vi "Frequency Linearization SubVI.vi"(8 "Scale factor":dbl(slide)=0.5 scale=0.01..1.0, 9 "#Medie":i32=20, 10 "Sketri Input":dbl[](array[numeric])=[2047.0, 2034.0, 2021.0, 2008.0, 1995.0, 1982.0, 1969.0, 1956.0, 1943.0, 1930.0, 1917.0, 1904.0, 1891.0, 1879.0, 1866.0, 1853.0, 1840.0, 1827.0, 1815.0, 1802.0, 1789.0, 1777.0, 1764.0, 1751.0, 1739.0, 1726.0, 1714.0, 1701.0, 1689.0, 1676.0, 1664.0, 1651.0, 1639.0, 1626.0, 1614.0, 1602.0, 1589.0, 1577.0, 1565.0, 1552.0, 1540.0, 1528.0, 1516.0, 1503.0, 1491.0, 1479.0, 1467.0, 1455.0, 1443.0, 1431.0, 1419.0, 1407.0, 1395.0, 1383.0, 1371.0, 1359.0, 1347.0, 1335.0, 1323.0, 1311.0, 1299.0, 1287.0, 1276.0, 1264.0, 1252.0, 1240.0, 1229.0, 1217.0, 1205.0, 1194.0, 1182.0, 1170.0, 1159.0, 1147.0, 1136.0, 1124.0, 1113.0, 1101.0, 1090.0, 1078.0, 1067.0, 1055.0, 1044.0, 1033.0, 1021.0, 1010.0, 999.0, 987.0, 976.0, 965.0, 954.0, 942.0, 931.0, 920.0, 909.0, 898.0, 887.0, 876.0, 865.0, 854.0, 843.0, 832.0, 821.0, 810.0, 799.0, 788.0, 777.0, 766.0, 755.0, 744.0, 734.0, 723.0, 712.0, 701.0, 691.0, 685.0, 679.0, 674.0, 665.0, 658.0, 652.0, 647.0, 640.0, 634.0, 628.0, 618.0, 612.0, 605.0, 600.0, 594.0, 587.0, 582.0, 575.0, 570.0, 564.0, 559.0, 553.0, 548.0, 542.0, 537.0, 531.0, 525.0, 520.0, 514.0, 509.0, 503.0, 497.0, 492.0, 486.0, 480.0, 475.0, 469.0, 463.0, 458.0, 452.0, 446.0, 441.0, 435.0, 429.0, 423.0, 417.0, 411.0, 406.0, 400.0, 395.0, 389.0, 383.0, 377.0, 372.0, 366.0, 360.0, 355.0, 349.0, 344.0, 338.0, 333.0, 328.0, 322.0, 317.0, 311.0, 306.0, 300.0, 295.0, 289.0, 284.0, 278.0, 273.0, 268.0, 262.0, 257.0, 251.0, 246.0, 240.0, 235.0, 229.0, 224.0, 219.0, 213.0, 208.0, 202.0, 197.0, 191.0, 186.0, 181.0, 175.0, 170.0, 164.0, 159.0, 154.0, 148.0, 143.0, 137.0, 132.0, 127.0, 121.0, 116.0, 110.0, 105.0, 100.0, 94.0, 89.0, 84.0, 78.0, 73.0, 67.0, 62.0, 57.0, 51.0, 46.0, 41.0, 35.0, 30.0, 25.0, 19.0, 14.0, 8.0, 3.0, -3.0, -8.0, -13.0, -18.0, -24.0, -29.0, -35.0, -40.0, -45.0, -51.0, -56.0, -62.0, -67.0, -72.0, -78.0, -83.0, -88.0, -94.0, -99.0, -104.0, -110.0, -115.0, -120.0, -126.0, -131.0, -137.0, -142.0, -147.0, -153.0, -158.0, -163.0, -169.0, -174.0, -179.0, -185.0, -190.0, -195.0, -201.0, -206.0, -211.0, -217.0, -222.0, -227.0, -233.0, -238.0, -243.0, -249.0, -254.0, -259.0, -265.0, -270.0, -275.0, -281.0, -286.0, -291.0, -297.0, -302.0, -307.0, -313.0, -318.0, -323.0, -329.0, -334.0, -339.0, -345.0, -350.0, -355.0, -361.0, -366.0, -371.0, -377.0, -382.0, -387.0, -393.0, -398.0, -403.0, -408.0, -414.0, -419.0, -424.0, -430.0, -435.0, -440.0, -446.0, -451.0, -456.0, -462.0, -467.0, -472.0, -478.0, -483.0, -488.0, -494.0, -499.0, -504.0, -510.0, -515.0, -520.0, -526.0, -531.0, -536.0, -541.0, -547.0, -552.0, -557.0, -563.0, -568.0, -573.0, -579.0, -584.0, -589.0, -594.0, -600.0, -605.0, -610.0, -616.0, -621.0, -626.0, -631.0, -637.0, -642.0, -647.0, -652.0, -658.0, -663.0, -668.0, -673.0, -679.0, -684.0, -689.0, -695.0, -700.0, -705.0, -710.0, -716.0, -721.0, -726.0, -731.0, -737.0, -742.0, -747.0, -753.0, -758.0, -763.0, -768.0, -774.0, -779.0, -784.0, -789.0, -795.0, -800.0, -805.0, -811.0, -816.0, -821.0, -826.0, -832.0, -837.0, -842.0, -848.0, -853.0, -858.0, -864.0, -869.0, -874.0, -879.0, -885.0, -890.0, -895.0, -901.0, -906.0, -911.0, -916.0, -922.0, -927.0, -932.0, -938.0, -943.0, -948.0, -953.0, -959.0, -964.0, -969.0, -974.0, -980.0, -985.0, -990.0, -996.0, -1001.0, -1006.0, -1011.0, -1017.0, -1022.0, -1027.0, -1032.0, -1038.0, -1043.0, -1048.0, -1054.0, -1059.0, -1064.0, -1069.0, -1075.0, -1080.0, -1085.0, -1090.0, -1096.0, -1101.0, -1106.0, -1112.0, -1117.0, -1122.0, -1127.0, -1133.0, -1138.0, -1143.0, -1148.0, -1154.0, -1159.0, -1164.0, -1169.0, -1175.0, -1180.0, -1185.0, -1191.0, -1196.0, -1201.0, -1206.0, -1212.0, -1217.0, -1222.0, -1227.0, -1233.0, -1238.0, -1243.0, -1249.0, -1254.0, -1259.0, -1264.0, -1270.0, -1275.0, -1280.0, -1285.0, -1291.0, -1296.0, -1301.0, -1306.0, -1312.0, -1317.0, -1322.0, -1328.0, -1333.0, -1338.0, -1343.0, -1349.0, -1354.0, -1359.0, -1364.0, -1370.0, -1375.0, -1380.0, -1385.0, -1391.0, -1396.0, -1401.0, -1407.0, -1412.0, -1417.0, -1422.0, -1428.0, -1433.0, -1438.0, -1443.0, -1449.0, -1454.0, -1459.0, -1464.0, -1470.0, -1475.0, -1480.0, -1486.0, -1491.0, -1496.0, -1501.0, -1507.0, -1512.0, -1517.0, -1522.0, -1528.0, -1533.0, -1538.0, -1543.0, -1549.0, -1554.0, -1559.0, -1564.0, -1570.0, -1575.0, -1580.0, -1586.0, -1591.0, -1596.0, -1601.0, -1607.0, -1612.0, -1617.0, -1622.0, -1628.0, -1633.0, -1638.0, -1643.0, -1649.0, -1654.0, -1659.0, -1664.0, -1670.0, -1675.0, -1680.0, -1685.0, -1691.0, -1696.0, -1701.0, -1706.0, -1712.0, -1717.0, -1722.0, -1728.0, -1733.0, -1738.0, -1743.0, -1749.0, -1754.0, -1759.0, -1764.0, -1770.0, -1775.0, -1780.0, -1785.0, -1791.0, -1796.0, -1801.0, -1806.0, -1812.0, -1817.0, -1822.0, -1827.0, -1833.0, -1838.0, -1843.0, -1848.0, -1854.0, -1859.0, -1864.0, -1869.0, -1875.0, -1880.0, -1885.0, -1890.0, -1896.0, -1901.0, -1906.0, -1911.0, -1917.0, -1922.0, -1927.0, -1932.0, -1938.0, -1943.0, -1948.0, -1953.0, -1959.0, -1964.0, -1969.0, -1974.0, -1980.0, -1985.0, -1990.0, -1995.0, -2001.0, -2006.0, -2011.0, -2016.0, -2022.0, -2027.0, -2032.0, -2037.0, -2043.0, -2048.0, -2047.0, -2037.0, -2028.0, -2018.0, -2008.0, -1999.0, -1989.0, -1979.0, -1970.0, -1960.0, -1951.0, -1941.0, -1931.0, -1922.0, -1912.0, -1903.0, -1893.0, -1884.0, -1874.0, -1865.0, -1855.0, -1846.0, -1836.0, -1827.0, -1817.0, -1808.0, -1798.0, -1789.0, -1779.0, -1770.0, -1761.0, -1751.0, -1742.0, -1732.0, -1723.0, -1714.0, -1704.0, -1695.0, -1686.0, -1676.0, -1667.0, -1658.0, -1648.0, -1639.0, -1630.0, -1621.0, -1611.0, -1602.0, -1593.0, -1584.0, -1575.0, -1565.0, -1556.0, -1547.0, -1538.0, -1529.0, -1520.0, -1510.0, -1501.0, -1492.0, -1483.0, -1474.0, -1465.0, -1456.0, -1447.0, -1438.0, -1429.0, -1420.0, -1411.0, -1402.0, -1393.0, -1384.0, -1375.0, -1366.0, -1357.0, -1348.0, -1339.0, -1330.0, -1321.0, -1312.0, -1303.0, -1294.0, -1285.0, -1277.0, -1268.0, -1259.0, -1250.0, -1241.0, -1232.0, -1224.0, -1215.0, -1206.0, -1197.0, -1188.0, -1180.0, -1171.0, -1162.0, -1153.0, -1145.0, -1136.0, -1127.0, -1119.0, -1110.0, -1101.0, -1093.0, -1084.0, -1075.0, -1067.0, -1058.0, -1049.0, -1041.0, -1032.0, -1024.0, -1015.0, -1007.0, -998.0, -989.0, -981.0, -972.0, -964.0, -955.0, -909.0, -902.0, -894.0, -872.0, -865.0, -858.0, -850.0, -843.0, -836.0, -781.0, -774.0, -747.0, -740.0, -734.0, -727.0, -720.0, -714.0, -707.0, -700.0, -693.0, -687.0, -679.0, -672.0, -654.0, -647.0, -639.0, -632.0, -625.0, -619.0, -608.0, -601.0, -595.0, -588.0, -582.0, -575.0, -568.0, -562.0, -555.0, -549.0, -542.0, -535.0, -529.0, -522.0, -515.0, -509.0, -502.0, -496.0, -489.0, -482.0, -476.0, -469.0, -462.0, -456.0, -449.0, -441.0, -435.0, -427.0, -420.0, -413.0, -407.0, -401.0, -395.0, -387.0, -381.0, -373.0, -367.0, -361.0, -355.0, -349.0, -343.0, -337.0, -330.0, -324.0, -318.0, -312.0, -306.0, -300.0, -294.0, -288.0, -282.0, -276.0, -269.0, -263.0, -257.0, -251.0, -245.0, -239.0, -233.0, -227.0, -221.0, -215.0, -209.0, -203.0, -197.0, -191.0, -185.0, -179.0, -173.0, -167.0, -161.0, -155.0, -149.0, -143.0, -137.0, -131.0, -125.0, -119.0, -113.0, -107.0, -101.0, -95.0, -89.0, -83.0, -77.0, -71.0, -65.0, -59.0, -54.0, -48.0, -42.0, -36.0, -30.0, -23.0, -17.0, -11.0, -6.0, -0.0, 6.0, 13.0, 19.0, 25.0, 31.0, 37.0, 42.0, 48.0, 55.0, 61.0, 66.0, 72.0, 78.0, 84.0, 89.0, 95.0, 101.0, 106.0, 112.0, 118.0, 124.0, 129.0, 135.0, 141.0, 146.0, 152.0, 157.0, 163.0, 169.0, 174.0, 180.0, 186.0, 191.0, 197.0, 203.0, 208.0, 214.0, 219.0, 225.0, 231.0, 236.0, 242.0, 247.0, 253.0, 259.0, 264.0, 270.0, 275.0, 281.0, 287.0, 292.0, 298.0, 303.0, 309.0, 315.0, 320.0, 326.0, 331.0, 337.0, 343.0, 348.0, 354.0, 359.0, 365.0, 371.0, 376.0, 382.0, 387.0, 393.0, 399.0, 404.0, 410.0, 416.0, 421.0, 427.0, 433.0, 438.0, 444.0, 449.0, 455.0, 461.0, 466.0, 472.0, 477.0, 483.0, 488.0, 494.0, 500.0, 505.0, 511.0, 517.0, 522.0, 528.0, 533.0, 539.0, 544.0, 550.0, 555.0, 561.0, 566.0, 572.0, 577.0, 583.0, 588.0, 594.0, 599.0, 604.0, 610.0, 615.0, 621.0, 626.0, 632.0, 637.0, 643.0, 648.0, 654.0, 659.0, 665.0, 670.0, 675.0, 681.0, 686.0, 692.0, 697.0, 703.0, 708.0, 714.0, 719.0, 725.0, 730.0, 735.0, 741.0, 746.0, 752.0, 757.0, 763.0, 768.0, 774.0, 779.0, 785.0, 790.0, 795.0, 801.0, 806.0, 812.0, 817.0, 823.0, 828.0, 834.0, 839.0, 844.0, 850.0, 855.0, 861.0, 866.0, 872.0, 877.0, 882.0, 888.0, 893.0, 899.0, 904.0, 910.0, 915.0, 920.0, 926.0, 931.0, 937.0, 942.0, 947.0, 953.0, 958.0, 964.0, 969.0, 974.0, 980.0, 985.0, 991.0, 996.0, 1001.0, 1007.0, 1012.0, 1018.0, 1023.0, 1028.0, 1034.0, 1039.0, 1045.0, 1050.0, 1055.0, 1061.0, 1066.0, 1071.0, 1077.0, 1082.0, 1088.0, 1093.0, 1098.0, 1104.0, 1109.0, 1114.0, 1120.0, 1125.0, 1130.0, 1136.0, 1141.0, 1146.0, 1152.0, 1157.0, 1162.0, 1168.0, 1173.0, 1178.0, 1184.0, 1189.0, 1194.0, 1200.0, 1205.0, 1210.0, 1216.0, 1221.0, 1226.0, 1232.0, 1237.0, 1242.0, 1248.0, 1253.0, 1258.0, 1264.0, 1269.0, 1274.0, 1280.0, 1285.0, 1290.0, 1296.0, 1301.0, 1306.0, 1312.0, 1317.0, 1322.0, 1328.0, 1333.0, 1338.0, 1344.0, 1349.0, 1355.0, 1360.0, 1365.0, 1371.0, 1376.0, 1381.0, 1387.0, 1392.0, 1397.0, 1403.0, 1408.0, 1413.0, 1419.0, 1424.0, 1429.0, 1434.0, 1440.0, 1445.0, 1450.0, 1456.0, 1461.0, 1466.0, 1472.0, 1477.0, 1482.0, 1488.0, 1493.0, 1498.0, 1504.0, 1509.0, 1514.0, 1520.0, 1525.0, 1530.0, 1536.0, 1541.0, 1546.0, 1552.0, 1557.0, 1562.0, 1567.0, 1573.0, 1578.0, 1583.0, 1589.0, 1594.0, 1599.0, 1605.0, 1610.0, 1615.0, 1621.0, 1626.0, 1631.0, 1636.0, 1642.0, 1647.0, 1652.0, 1658.0, 1663.0, 1668.0, 1674.0, 1679.0, 1684.0, 1689.0, 1695.0, 1700.0, 1705.0, 1711.0, 1716.0, 1721.0, 1727.0, 1732.0, 1737.0, 1742.0, 1748.0, 1753.0, 1758.0, 1764.0, 1769.0, 1774.0, 1779.0, 1785.0, 1790.0, 1795.0, 1801.0, 1806.0, 1811.0, 1816.0, 1822.0, 1827.0, 1832.0, 1837.0, 1843.0, 1848.0, 1853.0, 1859.0, 1864.0, 1869.0, 1874.0, 1880.0, 1885.0, 1890.0, 1895.0, 1901.0, 1906.0, 1911.0, 1917.0, 1922.0, 1927.0, 1932.0, 1938.0, 1943.0, 1948.0, 1953.0, 1959.0, 1964.0, 1969.0, 1974.0, 1980.0, 1985.0, 1990.0, 1995.0, 2001.0, 2006.0, 2011.0, 2016.0, 2022.0, 2027.0, 2032.0, 2037.0, 2043.0, 2048.0], 11 "Triangolo dritto":bool=TRUE) -> (0 "Second Signal (Last)":dbl[](graph), 1 "First Signal (Last)":dbl[](graph), 2 "Rising Std Dev %":dbl, 3 "Falling Std Dev %":dbl, 4 "Last Mean Freq Curve Falling":dbl[](graph), 6 "Last Mean Freq Curve Rising":dbl[](graph))   [LabVIEW 2014]
uses:
  <vilib>/rvi/interface/nirviOpenFPGA/nirviOpenFPGA.xnode
  <vilib>/rvi/interface/nirviMethod/nirviMethod.xnode
  <vilib>/FPGAPlugInAG/Dynamic/niLvFpga_ConfigureFifo_Dynamic.vi
  <vilib>/rvi/errors/niLvFpgaMergeErrorWithErrorCode.vi
  <vilib>/FPGAPlugInAG/Dynamic/niLvFpga_StartFifo_Dynamic.vi
  <vilib>/FPGAPlugInAG/Dynamic/niLvFpga_Run_Dynamic.vi
  <vilib>/FPGAPlugInAG/Dynamic/niLvFpga_Abort_Dynamic.vi
  <vilib>/rvi/interface/nirviCloseFPGA/nirviCloseFPGA.xnode
  <vilib>/rvi/interface/nirviReadWriteControl/nirviReadWriteControl.xnode
  <vilib>/rvi/interface/Simulation/niFpgaSimulationCallBeginRW.vi
  <vilib>/rvi/errors/niLvFpgaAdjustHostInterfaceError.vi
  <vilib>/FPGAPlugInAG/Dynamic/niLvFpga_ReadFifo_Dynamic.vi
  <vilib>/Platform/TimedLoop/XDataNode/XDataNode.xnode
  <vilib>/Platform/TimedLoop/XDataNode/nitl_modes.ctl
  <vilib>/Platform/TimedLoop/XDataNode/XDNodeRunTimeDep.lvlib
  <vilib>/Platform/TimedLoop/XDataNode/wakeup.ctl
  <vilib>/Platform/TimedLoop/XDataNode/timing_clust.ctl
  <vilib>/FPGAPlugInAG/Dynamic/niLvFpga_Reset_Dynamic.vi
  NiFpgaLv.dll
  <vilib>/Utility/error.llb/Error Cluster From Error Code.vi
  <vilib>/FPGAPlugInAG/Dynamic/niLvFpga_Close_Dynamic.vi
  FPGA Target/Test VIs/Double FFT Mesurament Test.vi
panel:
  in  "Acrive  Smooth":bool
  out "Complete SkewTri":dbl[](graph)
  out "2) Tri edge RISING":dbl[](graph)
  out "1) Tri edge FALLING":dbl[](graph)
  out "1) Ext Mean Freq Curve":dbl[](graph)
  out "2) Ext Mean Freq Curve":dbl[](graph)
  out "2) Mean Freq Curve Rising":dbl[](graph)
  out "1) Mean Freq Curve Falling":dbl[](graph)
  out "2) Freq curve":dbl[](graph)
  out "1) Freq curve":dbl[](graph)
  in  "FFT Sliding Win Size":i32=128
  out "1) SmoothSubSig":dbl[](graph)
  out "2) SmoothSubSig":dbl[](graph)
  in  "Acrive Fit":bool=TRUE
  in  "Poly Order":i32=3
  in  "Side points":i32=13
  in  "Poly Grade":dbl=5.0
  out "2) Signal&Fit 2":dbl[][](graph)
  out "1) Signal&Fit":dbl[][](graph)
  out "Current Sig lin":i32
  in  "Acrive Linearization":bool=TRUE
  in  "?":bool
  out "maxbin_secondFFT":i32
  out "maxbin_firstFFT":i32
  out "f_rise":dbl
  out "f_fall":dbl
  out "f_mean":dbl
  out "Velocity (m/s)":dbl
  out "Distance (m)":dbl
  in  "Initial Latency points":u32(slide) scale=0.0..1249.0
  out "Second FFT (bin)":dbl[](graph)
  out "Second Signal (points) - Rising Triangular":dbl[](graph)
  out "First FFT (bin)":dbl[](graph)
  out "First Signal (points) - Falling Triangular":dbl[](graph)
  in  "Windowing":T1(ring)
  in  "first bin":i32=5
  in  "last bin":i32=255
  in  "lower limit 2":u32(slide)=738 scale=625.0..738.0
  in  "lower limit 1":u32(slide)=113 scale=0.0..113.0
  # "OFFLINE parameters"
  # "Triangolo storto\nda costante"
  # "Max Detection FFT bin range"
  # "ONLINE parameters"
  # "Se la sottrazione del fondo non è eseguita su FPGA.\n Attivarla per eseguirla lato RT"
  # "Smoothing (S-G Params)"
  # "Fitting"
  # "ONLY POWER OF 2"
  # "Min: 2 Max: 256 (2, 4, 8, 16, 32, 64, 128, 256)"
  # "LINEARIZATION FINAL RESULTS"
  # "%"
  # "%"
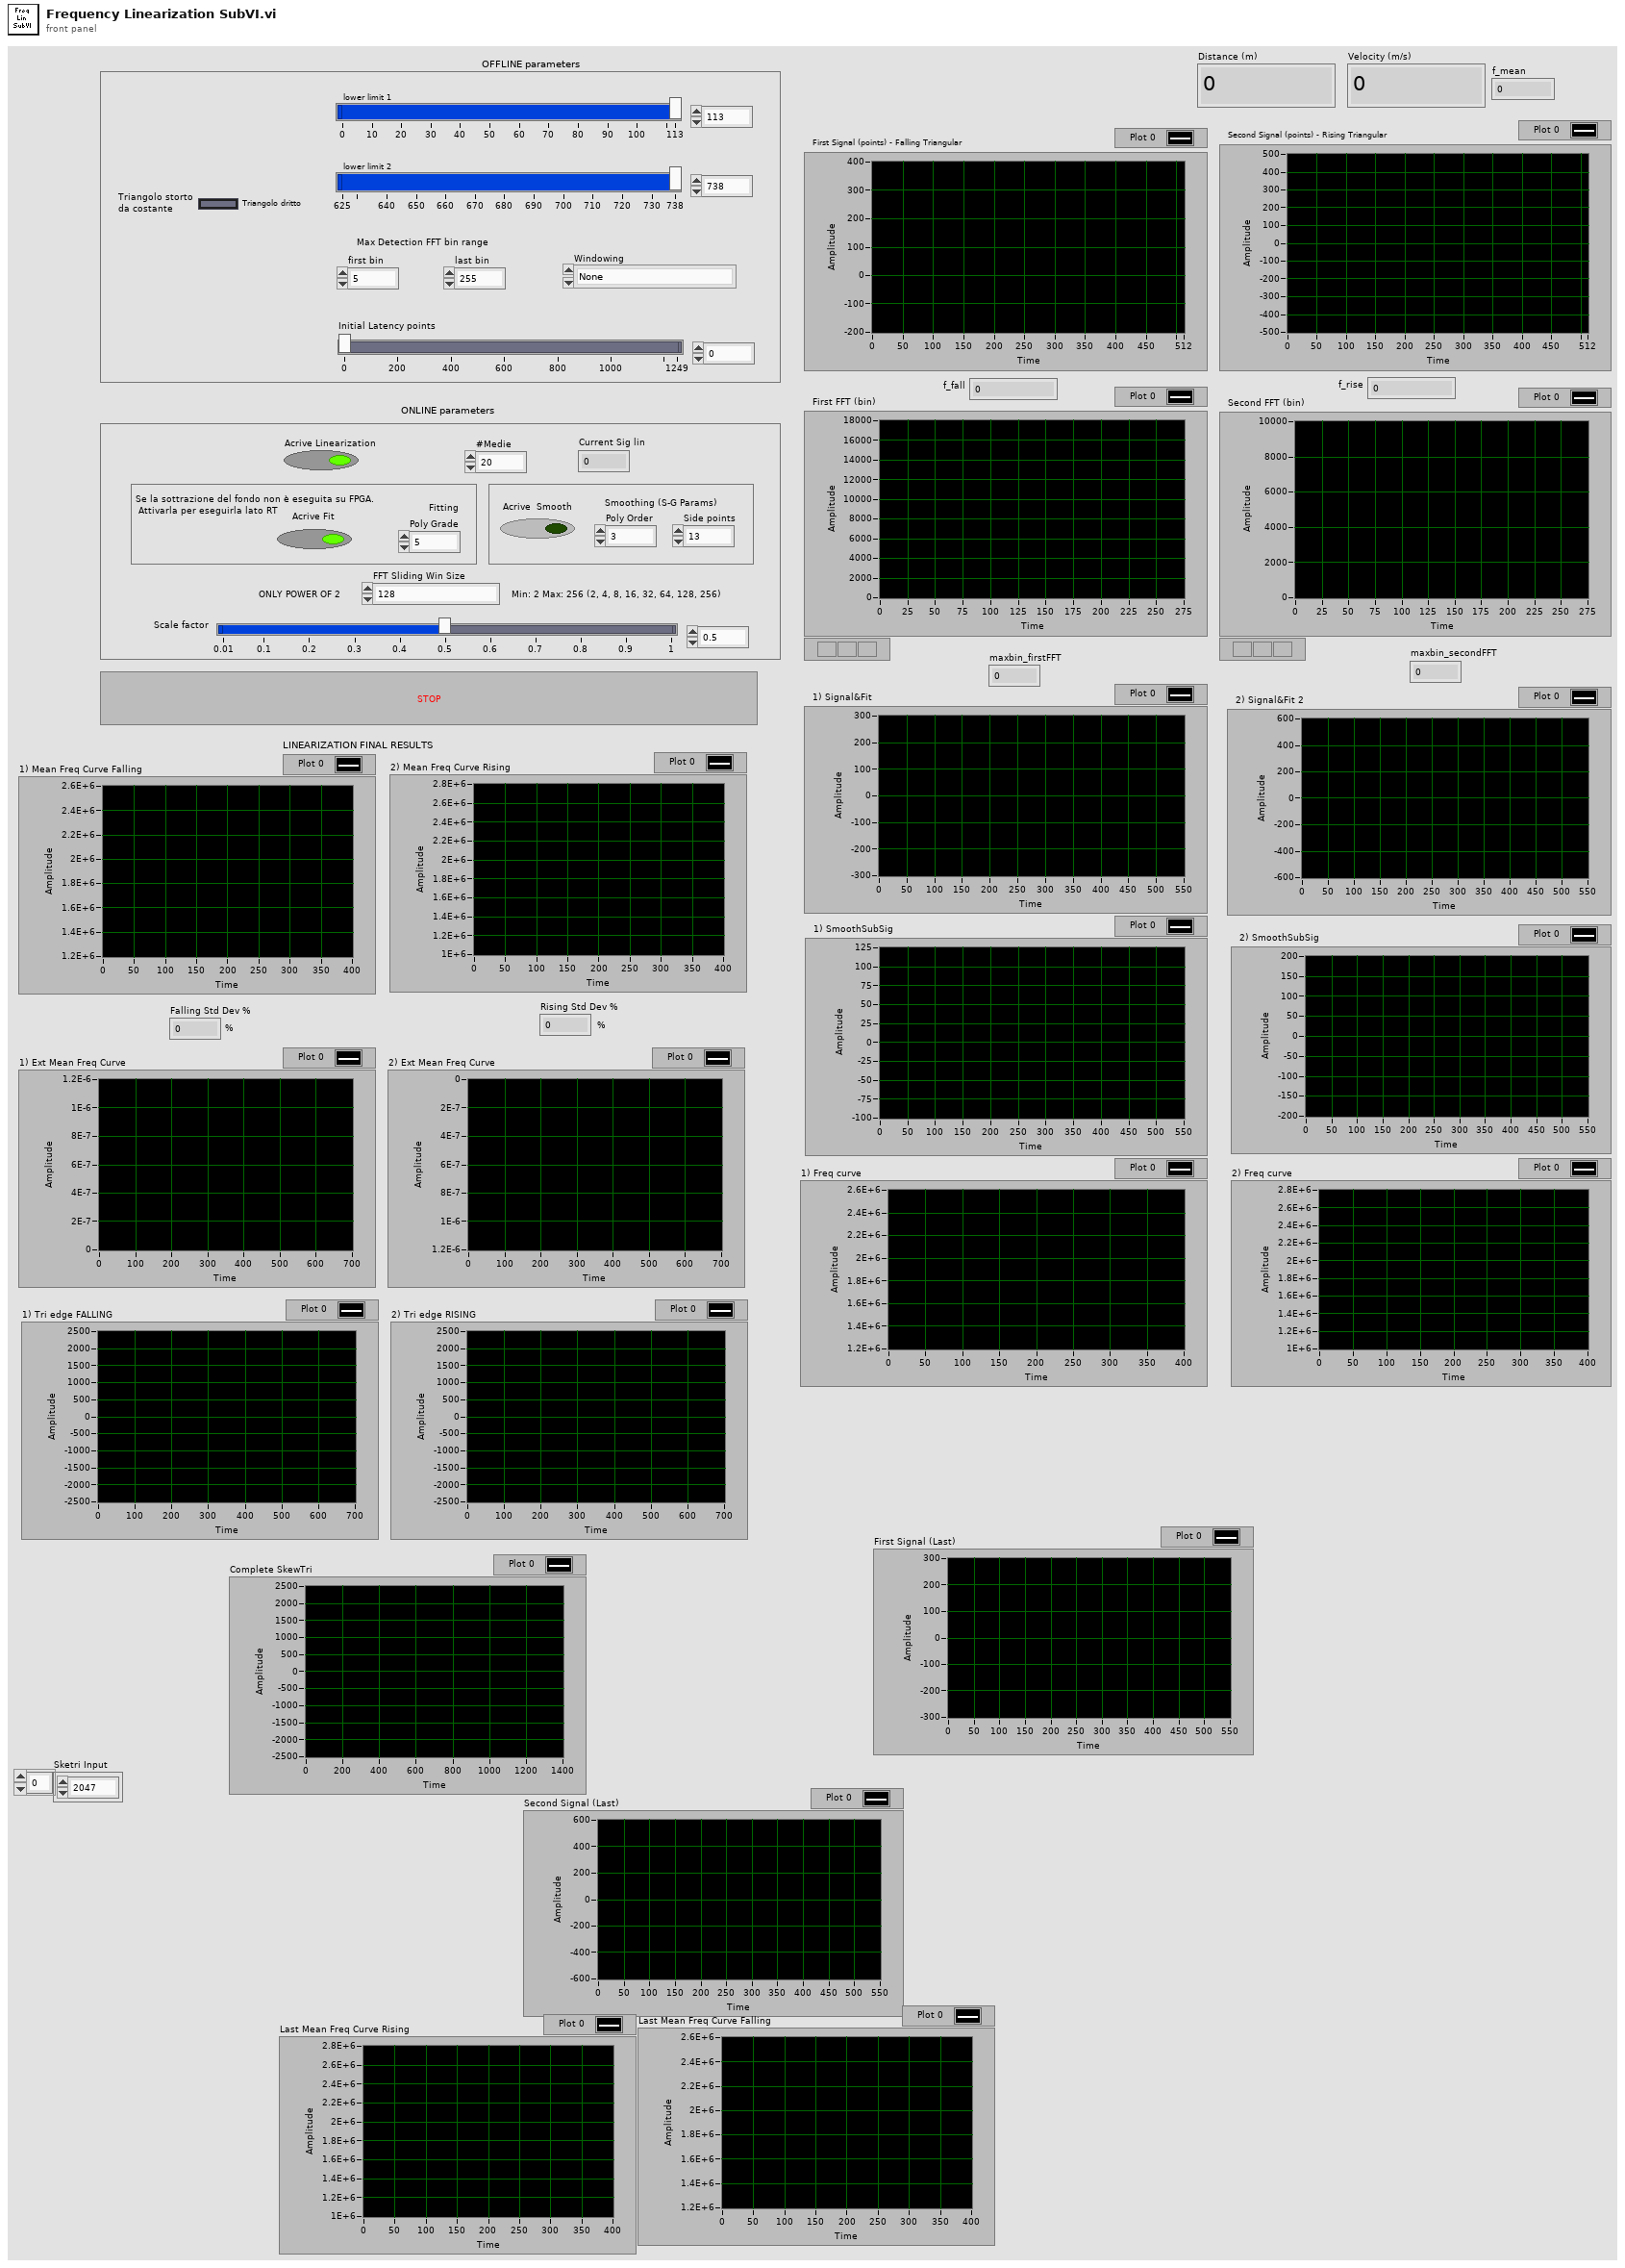
[diagram p1: front panel]
types:
  T1 = enum16{"None", "Hanning", "Hamming", "Blackman", "Blackman-Harris"}
  T2 = typedef "XDNodeRunTimeDep.lvlib/timing_clust.ctl" = cluster{"Expected End [f-1]":u64, "Actual End [f-1]":u64, "Finished Late? [f-1]":bool, "Expected End [i-1]":u64, "Actual End [i-1]":u64, "Finished Late? [i-1]":bool, "Expected Start [i]":u64, "Actual Start [i]":u64, "Expected Start [f]":u64, "Actual Start [f]":u64, "Source Name":string, "Structure Name":string, "Period":i64, "Deadline":i64, "Offset":i64, "Start":i64, "Priority":i32, "Timeout":i32, "Mode":T3, "Wakeup Reason":T4, "Error":errorcluster, "Source Type":string, "Secondary Source Type":string, "Global End Time":u64, "Global Start Time":u64, "Frame Duration":u64, "Iteration Duration":u64, "Assigned CPU":i32, "I/O Scan Engine Mode":u32}
  T3 = typedef "XDNodeRunTimeDep.lvlib/nitl_modes.ctl" = enum32{"No Change", "Process missed periods, maintain original phase", "Discard missed periods, maintain original phase", "Process missed periods, ignore original phase", "Discard missed periods, ignore original phase"}
  T4 = typedef "XDNodeRunTimeDep.lvlib/wakeup.ctl" = enum32{"Normal", "Aborted", "Asynchronous wakeup", "Timing source error", "Timed loop error", "Timeout"}
  T5 = typedef "NI_Matrix.lvlib/RealMatrix.ctl" = dbl[][]
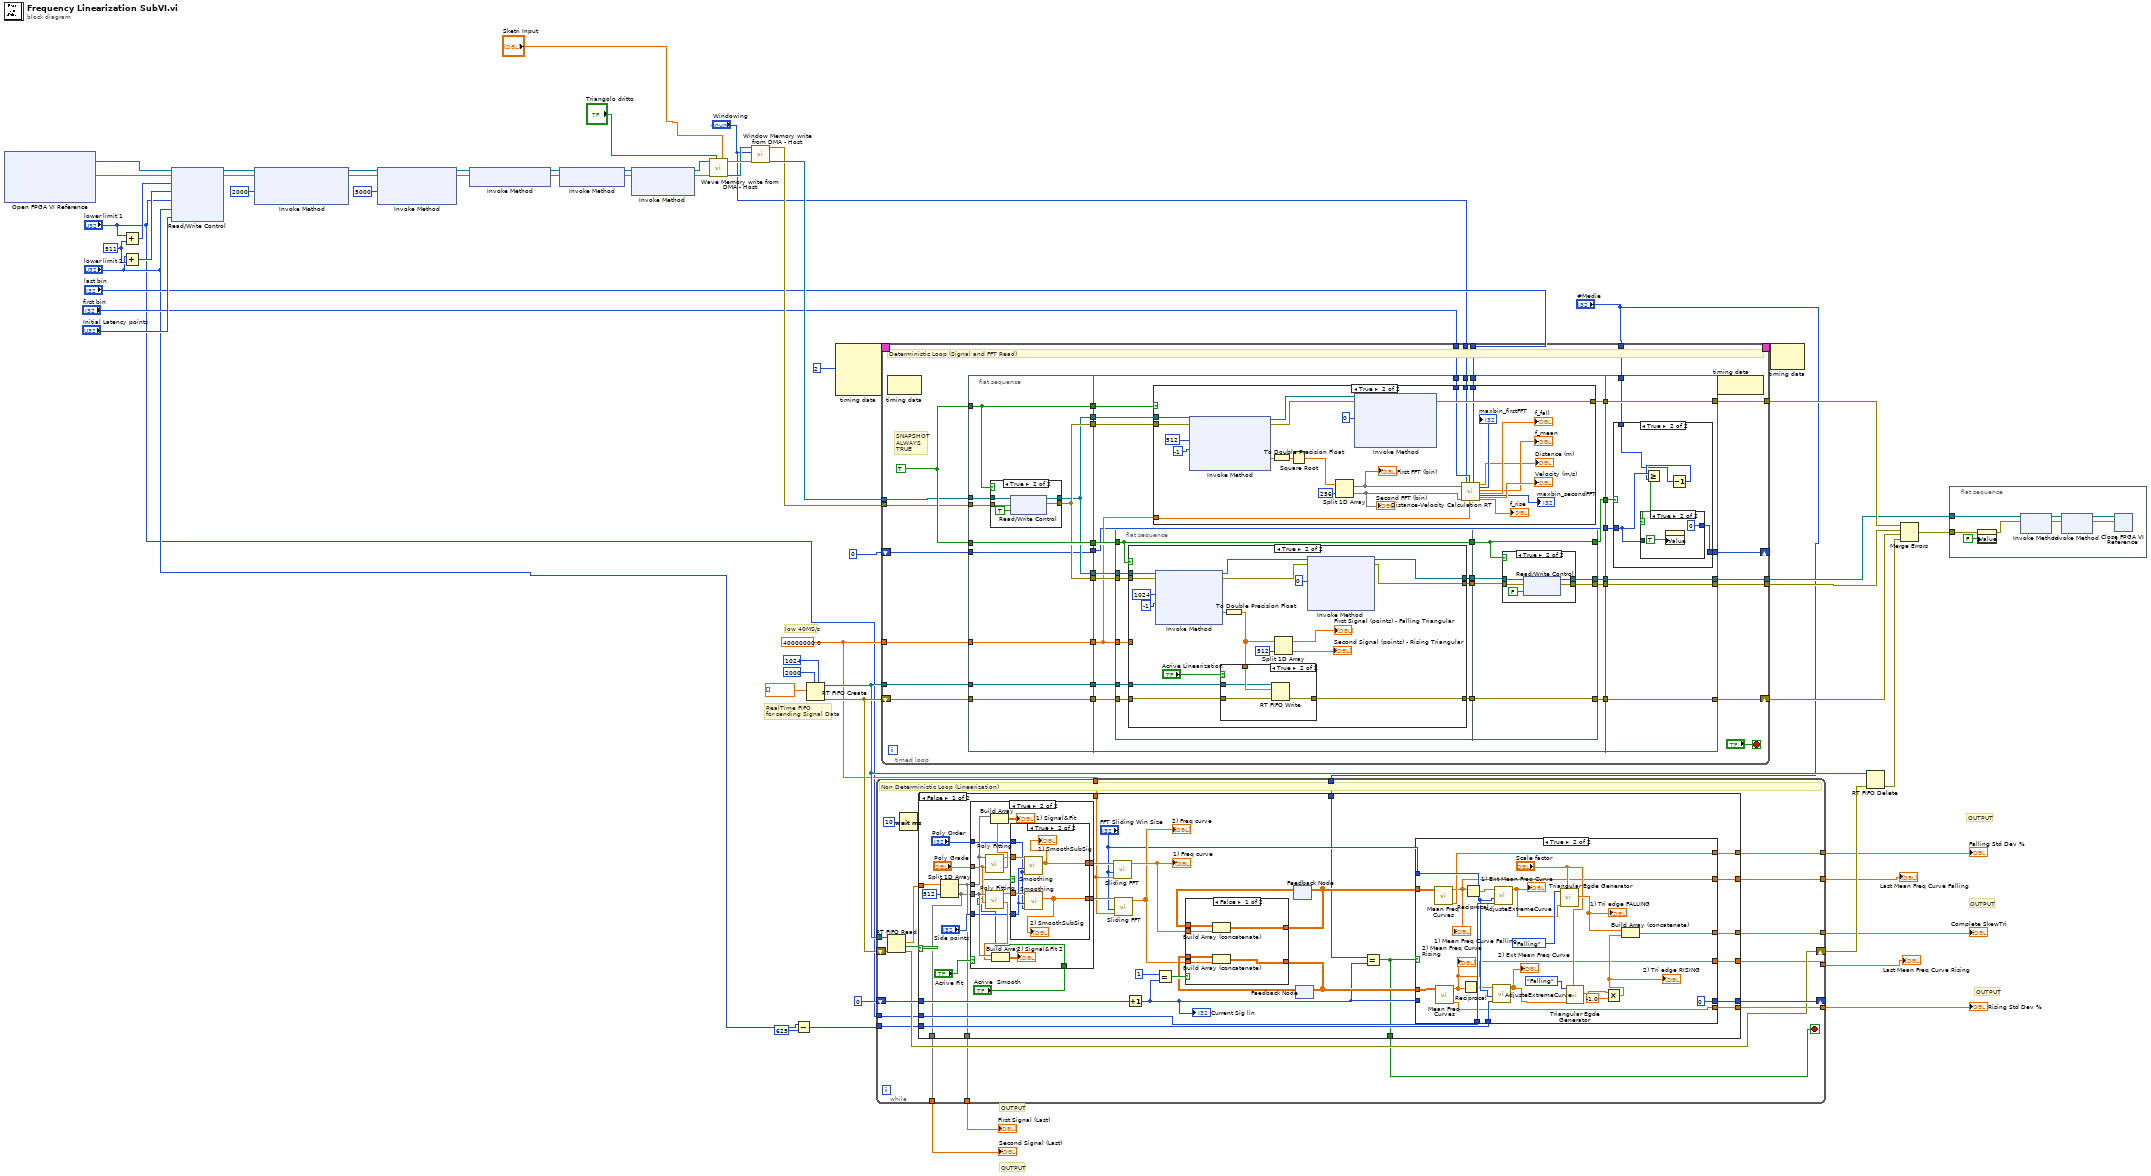
[diagram p0: block diagram]
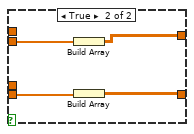
[diagram p5: hidden frame]
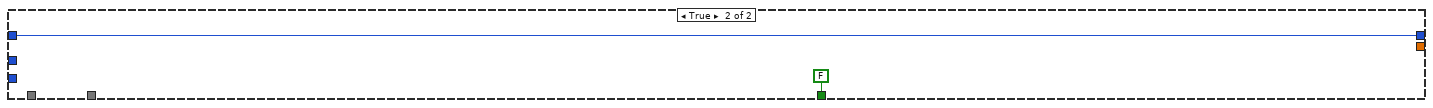
[diagram p6: hidden frame]
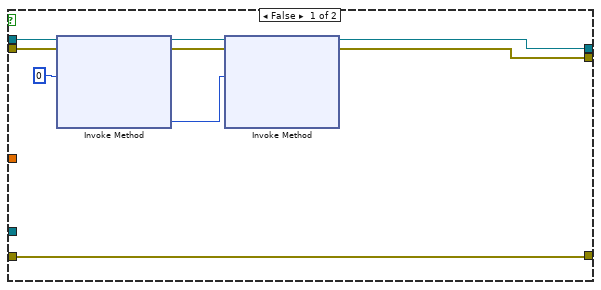
[diagram p8: hidden frame]
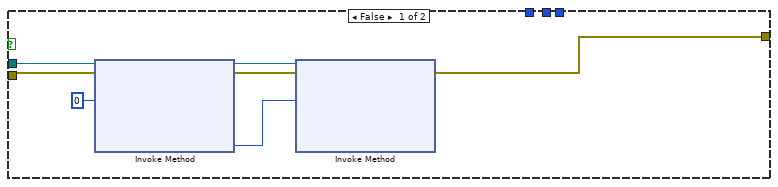
[diagram p11: hidden frame]
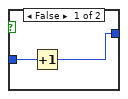
[diagram p13: hidden frame]
diagram:
  w57 = u32 511 ("y")
  w12 = 40000000.0 ("Sample Rate (S/s)")
  # "OUTPUT"
  # "OUTPUT"
  # "OUTPUT"
  # "OUTPUT"
  # "OUTPUT"
  # "RealTime FIFO \nfor sending Signal Data"
  # "low 40MS/s"
  n1 = xnode "Open FPGA VI Reference"() -> ("FPGA VI Reference Out"=w56:refnum<k20>, "error out"=w55:errorcluster)  [unwired: 2 in]
  n2 = Add(x="lower limit 1", y=w57) -> (x+y=w59:u32)
  n3 = Add(x="lower limit 2", y=w57) -> (x+y=w58:u32)
  n4 = xnode "Read/Write Control"("FPGA VI Reference In"=w56, "error in"=w55, "upper limit 1"=w59, "upper limit 2"=w58, "lower limit 1"="lower limit 1", "lower limit 2"="lower limit 2", "Latency points"="Initial Latency points") -> ("FPGA VI Reference Out"=w52:refnum<k20>, "error out"=w51:errorcluster)
  n5 = xnode "Invoke Method"("FPGA VI Reference In"=w52, "error in"=w51, "Requested Depth"=u32 2000) -> ("FPGA VI Reference Out"=w30:refnum<k20>, "error out"=w31:errorcluster)  [unwired: 1 out]
  n6 = xnode "Invoke Method"("FPGA VI Reference In"=w30, "error in"=w31, "Requested Depth"=u32 5000) -> ("FPGA VI Reference Out"=w44:refnum<k20>, "error out"=w45:errorcluster)  [unwired: 1 out]
  n7 = xnode "Invoke Method"("FPGA VI Reference In"=w44, "error in"=w45) -> ("FPGA VI Reference Out"=w28:refnum<k20>, "error out"=w29:errorcluster)
  n8 = xnode "Invoke Method"("FPGA VI Reference In"=w28, "error in"=w29) -> ("FPGA VI Reference Out"=w42:refnum<k20>, "error out"=w43:errorcluster)
  n9 = xnode "Invoke Method"("FPGA VI Reference In"=w42, "error in"=w43) -> ("FPGA VI Reference Out"=w48:refnum<k20>, "error out"=w47:errorcluster)  [unwired: 1 in]
  n10 = call "Wave Memory write from DMA - Host.vi"("Custom Triangular Signal (fal-ris)"="Sketri Input", "Triangolo dritto?"="Triangolo dritto", "error in"=w47, "FPGA VI Reference In"=w48) -> ("FPGA VI Reference Out"=w33:refnum<k20>, "error out"=w46:errorcluster)  [unwired: 5 in, 1 out]
  n11 = call "Window Memory write from DMA - Host.vi"("error in"=w46, "Enum"="Windowing", "FPGA VI Reference In"=w33) -> ("FPGA VI Reference Out"=w54:refnum<k20>, "error out"=w53:errorcluster)  [unwired: 5 in, 2 out]
  n12 = Subtract(x="lower limit 2", y=u32 625) -> (x-y=w14:u32)
  n13 = RT FIFO Create(1:dbl[] [] ("double precision float"), 4:u32 2000 ("size (10)"), 6:u32 1024 ("elements in array (1)")) -> (8:w20:refnum<k33>, 11:w22:errorcluster)  [unwired: 5 in, 1 out]
  n14 = node-c288(i64 2 ("Period")) -> (w41:T2)  [unwired: 3 in]
  n15 = while {
    shift-right: [w72] -> w19
    shift-left: w22 -> [w74]
    tunnel: w20 -> [w78]
    shift-right: [w73] -> _
    shift-left: 0 -> [w77]
    tunnel: "lower limit 1" -> [w69]
    tunnel: w14 -> [w70]
    tunnel: w12 -> [w71]
    tunnel: [w68] -> w8
    tunnel: [w67] -> w7
    tunnel: [w66] -> w6
    tunnel: [w65] -> w5
    tunnel: [w64] -> w4
    tunnel: "#Medie" -> [w63]
    tunnel: [w61] -> w2
    tunnel: [w60] -> w1
    stop <- w62 stop-if-true
    # "Non Deterministic Loop (Linearization)"
    n16 = RT FIFO Read(0:w78, 3:w74) -> (9:w76:dbl[], 10:w75:bool, 11:w72:errorcluster)  [unwired: 2 in, 2 out]
    n17 = Wait (ms)(milliseconds to wait=u32 10 ("millisecond multiple")) -> ()  [unwired: 1 out]
    n18 = case shown="False" w75 {
      tunnel: w77 -> [w112 w171]
      tunnel: [w102 w171] -> w73
      tunnel: w76 -> [w110 _]
      tunnel: w71 -> [w95 _]
      tunnel: w70 -> [w92 _]
      tunnel: w69 -> [w91 _]
      tunnel: [w88 _] -> w68
      tunnel: [w87 _] -> w67
      tunnel: [w86 _] -> w66
      tunnel: [w85 _] -> w65
      tunnel: [w84 _] -> w64
      tunnel: w63 -> [w83 _]
      tunnel: [w82 FALSE] -> w62
      tunnel: [w81 _] -> w61
      tunnel: [w80 _] -> w60
      frame False {
        n19 = Split 1D Array(array=w110, index=512) -> (first subarray=w85:dbl[], second subarray=w84:dbl[])
        n20 = case shown="True" "Acrive Fit" {
          tunnel: w85 -> [w114 w128]
          tunnel: w84 -> [w113 w124]
          tunnel: "Poly Grade" -> [_ w120]
          tunnel: "Side points" -> [_ w119]
          tunnel: "Poly Order" -> [_ w118]
          tunnel: [w113 w117] -> w96
          tunnel: [w114 w115] -> w97
          tunnel: "Acrive  Smooth" -> [_ w116]
          frame False {
          }
          frame True {
            n21 = call "Poly Fitting.vi"("Poly Grade"=w120, "Signal"=w128) -> ("Poly Signal"=w127:dbl[], "SubtractedSignal"=w122:dbl[])  [unwired: 8 in]
            n22 = call "Poly Fitting.vi"("Poly Grade"=w120, "Signal"=w124) -> ("Poly Signal"=w123:dbl[], "SubtractedSignal"=w121:dbl[])  [unwired: 8 in]
            n23 = Build Array(w128, w127) -> (→"1) Signal&Fit":dbl[][])
            n24 = Build Array(w124, w123) -> (→"2) Signal&Fit 2":dbl[][])
            n25 = case shown="True" w116 {
              tunnel: w122 -> [w130 w136]
              tunnel: w121 -> [w129 w135]
              tunnel: w119 -> [_ w134]
              tunnel: w118 -> [_ w133]
              tunnel: [w129 w132] -> w117
              tunnel: [w130 w131] -> w115
              frame False {
              }
              frame True {
                n26 = call "Smoothing.vi"("polynomial order"=w133, "side points"=w134, "SubtractedSignal"=w136) -> ("SubSmoothSignal"=w131:dbl[])  [unwired: 8 in]
                "1) SmoothSubSig" <- w131
                n27 = call "Smoothing.vi"("polynomial order"=w133, "side points"=w134, "SubtractedSignal"=w135) -> ("SubSmoothSignal"=w132:dbl[])  [unwired: 8 in]
                "2) SmoothSubSig" <- w132
              }
            }
          }
        }
        n28 = call "Sliding FFT.vi"("Sample Freq"=w95, "FFT Win Size"="FFT Sliding Win Size", "SubSmoothSignal"=w97) -> ("Freq samples"=w94:dbl[])  [unwired: 7 in, 1 out]
        "1) Freq curve" <- w94
        n29 = call "Sliding FFT.vi"("Sample Freq"=w95, "FFT Win Size"="FFT Sliding Win Size", "SubSmoothSignal"=w96) -> ("Freq samples"=w93:dbl[])  [unwired: 7 in, 1 out]
        "2) Freq curve" <- w93
        n30 = Increment(x=w112) -> (x+1=w103:i32)
        "Current Sig lin" <- w103
        n31 = Equal?(x=1, y=w103) -> (x = y?=w108:bool)
        n32 = feedback #1() -> (w107:T5)  [unwired: 1 in]
        n33 = feedback #2() -> (w106:T5)  [unwired: 1 in]
        n34 = case shown="False" w108 {
          tunnel: w93 -> [w164 w167]
          tunnel: w94 -> [w165 w169]
          tunnel: [w163 w166] -> w104
          tunnel: [w162 w168] -> w105
          tunnel: w107 -> [w161 _]
          tunnel: w106 -> [w160 _]
          frame False {
            n35 = Build Array (concatenate)(w161, w165) -> (w162:T5)
            n36 = Build Array (concatenate)(w160, w164) -> (w163:T5)
          }
          frame True {
            n37 = Build Array(w169) -> (w168:T5)
            n38 = Build Array(w167) -> (w166:T5)
          }
        }
        n39 = feedback-in #1(w105) -> ()
        n40 = feedback-in #2(w104) -> ()
        n41 = Equal?(x=w83, y=w103) -> (x = y?=w82:bool)
        n42 = case shown="True" w82 {
          tunnel: w105 -> [_ w158]
          tunnel: w104 -> [_ w157]
          tunnel: w103 -> [w137 _]
          tunnel: [w137 0] -> w102
          tunnel: w92 -> [_ w153]
          tunnel: w91 -> [_ w152]
          tunnel: "FFT Sliding Win Size" -> [_ w151]
          tunnel: [_ w142] -> w88
          tunnel: [_ w141] -> w87
          tunnel: [_ w140] -> w86
          tunnel: [_ w139] -> w81
          tunnel: [_ w138] -> w80
          frame False {
          }
          frame True {
            n43 = call "Mean Freq Curves.vi"("Set of Freq samples"=w158) -> ("StdDev%"=w141:dbl, "Mean Freq Curve"=w139:dbl[])  [unwired: 9 in]
            "1) Mean Freq Curve Falling" <- w139
            n44 = call "Mean Freq Curves.vi"("Set of Freq samples"=w157) -> ("StdDev%"=w140:dbl, "Mean Freq Curve"=w138:dbl[])  [unwired: 9 in]
            "2) Mean Freq Curve Rising" <- w138
            n45 = Reciprocal(x=w138) -> (1/x=w148:dbl[])
            n46 = Reciprocal(x=w139) -> (1/x=w147:dbl[])
            n47 = call "AdjusteExtremeCurve.vi"("Init Bins Discarded"=w153, "FFT Size Window"=w151, "Freq sample"=w148) -> ("Extended Freq Sample"=w149:dbl[])  [unwired: 8 in]
            "2) Ext Mean Freq Curve" <- w149
            n48 = call "AdjusteExtremeCurve.vi"("Init Bins Discarded"=w152, "FFT Size Window"=w151, "Freq sample"=w147) -> ("Extended Freq Sample"=w150:dbl[])  [unwired: 8 in]
            "1) Ext Mean Freq Curve" <- w150
            n49 = call "Triangular Egde Generator.vi"("fattore"="Scale factor", "Sample values"=w150, "Triangular edge"=enum16{"Rising", "Falling"}."Falling") -> ("Skew Triangular"=w154:dbl[])  [unwired: 8 in]
            "1) Tri edge FALLING" <- w154
            n50 = call "Triangular Egde Generator.vi"("fattore"="Scale factor", "Sample values"=w149, "Triangular edge"=enum16{"Rising", "Falling"}."Falling") -> ("Skew Triangular"=w145:dbl[])  [unwired: 8 in]
            n51 = Multiply(x=w145, y=-1.0) -> (x*y=w144:dbl[])
            "2) Tri edge RISING" <- w144
            n52 = Build Array (concatenate)(w154, w144) -> (w142:dbl[])
          }
        }
      }
      frame True {
      }
    }
  }
  "Complete SkewTri" <- w8
  "Falling Std Dev %" <- w7
  "Rising Std Dev %" <- w6
  "First Signal (Last)" <- w5
  "Second Signal (Last)" <- w4
  "Last Mean Freq Curve Falling" <- w2
  "Last Mean Freq Curve Rising" <- w1
  n53 = timed-loop {
    tunnel: w54 -> [w199]
    tunnel: w53 -> [w200]
    tunnel: [w202] -> w38
    tunnel: w12 -> [w204]
    tunnel: [w203] -> w37
    timing: w41 -> [_]
    timing-out: [_] -> w40
    tunnel: "first bin" -> [w188]
    tunnel: "last bin" -> [w187]
    tunnel: [w185] -> w32
    tunnel: "Windowing" -> [w183]
    shift-right: [w177] -> w23
    shift-left: w22 -> [w179]
    tunnel: w20 -> [w181]
    shift-right: [w173] -> _
    shift-left: 0 -> [w175]
    tunnel: "#Medie" -> [w172]
    stop <- "?" stop-if-true
    w201 = TRUE ("Snapshot")
    # "SNAPSHOT\nALWAYS\nTRUE"
    # "Deterministic Loop (Signal and FFT Read)"
    n54 = node-c288() -> ()  [unwired: 1 in, 1 out]
    n55 = flat-sequence {
      tunnel: w199 -> [w212]
      tunnel: w200 -> [w213]
      tunnel: w201 -> [w210]
      tunnel: w201 -> [w215]
      tunnel: w204 -> [w216]
      tunnel: [w214] -> w198
      tunnel: [w216] -> w197
      tunnel: [w215] -> w196
      tunnel: [w210] -> w195
      tunnel: [w214] -> w194
      tunnel: [w211] -> w193
      tunnel: [w211] -> w192
      tunnel: [w209] -> w182
      tunnel: w181 -> [w209]
      tunnel: [w208] -> w180
      tunnel: w179 -> [w208]
      tunnel: [w207] -> w176
      tunnel: w175 -> [w207]
      tunnel: w198 -> [w241]
      tunnel: w197 -> [w229]
      tunnel: w196 -> [w235]
      tunnel: w195 -> [w238]
      tunnel: w194 -> [w237]
      tunnel: w193 -> [w236]
      tunnel: w192 -> [w242]
      tunnel: [w240] -> w191
      tunnel: [w239] -> w190
      tunnel: [w234] -> w189
      tunnel: w188 -> [w233]
      tunnel: w187 -> [w232]
      tunnel: [w231] -> w184
      tunnel: w183 -> [w230]
      tunnel: w182 -> [w228]
      tunnel: w180 -> [w227]
      tunnel: [w225] -> w178
      tunnel: w176 -> [w224]
      tunnel: [w224] -> w174
      tunnel: [w338] -> w202
      tunnel: [w339] -> w203
      tunnel: w191 -> [w339]
      tunnel: w190 -> [w338]
      tunnel: w189 -> [w337]
      tunnel: [w336] -> w185
      tunnel: w184 -> [w336]
      tunnel: [w335] -> w177
      tunnel: w178 -> [w335]
      tunnel: w174 -> [w334]
      tunnel: [w333] -> w173
      tunnel: w172 -> [w332]
      frame #0 {
        n56 = case shown="True" w210 {
          tunnel: [w217 w222] -> w214
          tunnel: w213 -> [w217 w221]
          tunnel: w212 -> [w218 w220]
          tunnel: [w218 w219] -> w211
          frame False {
          }
          frame True {
            n57 = xnode "Read/Write Control"("FPGA VI Reference In"=w220, "error in"=w221, "snapshot"=TRUE) -> ("FPGA VI Reference Out"=w219:refnum<k20>, "error out"=w222:errorcluster)
          }
        }
      }
      frame #1 {
        n58 = flat-sequence {
          tunnel: w242 -> [w254]
          tunnel: w241 -> [w253]
          tunnel: w229 -> [w252]
          tunnel: w235 -> [w249]
          tunnel: [w251] -> w245
          tunnel: [w250] -> w244
          tunnel: [w249] -> w243
          tunnel: w228 -> [w248]
          tunnel: w227 -> [w247]
          tunnel: [w246] -> w226
          tunnel: [w290] -> w239
          tunnel: w245 -> [w292]
          tunnel: w244 -> [w291]
          tunnel: w243 -> [w289]
          tunnel: [w289] -> w234
          tunnel: [w288] -> w231
          tunnel: [w287] -> w225
          tunnel: w226 -> [w287]
          frame #0 {
            n59 = case shown="True" w249 {
              tunnel: w254 -> [w262 w281]
              tunnel: w253 -> [w260 w280]
              tunnel: [w259 w273] -> w250
              tunnel: w252 -> [_ _]
              tunnel: [w256 w272] -> w251
              tunnel: w248 -> [_ w267]
              tunnel: w247 -> [w255 w266]
              tunnel: [w255 w265] -> w246
              frame False {
                n60 = xnode "Invoke Method"("FPGA VI Reference In"=w262, "error in"=w260, "Number of Elements"=u32 0) -> ("FPGA VI Reference Out"=w258:refnum<k20>, "error out"=w257:errorcluster, "Elements Remaining"=w261:u32)  [unwired: 1 in, 1 out]
                n61 = xnode "Invoke Method"("FPGA VI Reference In"=w258, "error in"=w257, "Number of Elements"=w261) -> ("FPGA VI Reference Out"=w256:refnum<k20>, "error out"=w259:errorcluster)  [unwired: 1 in, 2 out]
              }
              frame True {
                n62 = xnode "Invoke Method"("FPGA VI Reference In"=w281, "error in"=w280, "Number of Elements"=u32 1024, "Timeout (ms)"=-1) -> ("FPGA VI Reference Out"=w275:refnum<k20>, "error out"=w274:errorcluster, "Data"=w277:fxp<+/-,12,12>[])  [unwired: 1 out]
                n63 = To Double Precision Float(number=w277) -> (double precision float=w268:dbl[])
                n64 = case shown="True" "Acrive Linearization" {
                  tunnel: w268 -> [_ w286]
                  tunnel: w267 -> [_ w285]
                  tunnel: w266 -> [w282 w284]
                  tunnel: [w282 w283] -> w265
                  frame False {
                  }
                  frame True {
                    n65 = RT FIFO Write(0:w285, 1:w286, 3:w284) -> (11:w283:errorcluster)  [unwired: 2 in, 3 out]
                  }
                }
                n66 = Split 1D Array(array=w268, index=512) -> (first subarray=→"First Signal (points) - Falling Triangular":dbl[], second subarray=→"Second Signal (points) - Rising Triangular":dbl[])
                n67 = xnode "Invoke Method"("FPGA VI Reference In"=w275, "error in"=w274, "Number of Elements"=u32 0) -> ("FPGA VI Reference Out"=w272:refnum<k20>, "error out"=w273:errorcluster)  [unwired: 1 in, 2 out]
              }
            }
          }
          frame #1 {
            n68 = case shown="True" w289 {
              tunnel: [w294 w297] -> w290
              tunnel: w292 -> [w293 w298]
              tunnel: w291 -> [w294 w296]
              tunnel: [w293 w295] -> w288
              frame False {
              }
              frame True {
                n69 = xnode "Read/Write Control"("FPGA VI Reference In"=w298, "error in"=w296, "snapshot"=FALSE) -> ("FPGA VI Reference Out"=w295:refnum<k20>, "error out"=w297:errorcluster)
              }
            }
          }
        }
        n70 = case shown="True" w238 {
          tunnel: w236 -> [w305 w326]
          tunnel: w237 -> [w302 w327]
          tunnel: [w301 w325] -> w240
          tunnel: w233 -> [_ w312]
          tunnel: w232 -> [_ w313]
          tunnel: w230 -> [_ w309]
          tunnel: w229 -> [_ w307]
          frame False {
            n71 = xnode "Invoke Method"("FPGA VI Reference In"=w305, "error in"=w302, "Number of Elements"=u32 0) -> ("FPGA VI Reference Out"=w303:refnum<k20>, "error out"=w300:errorcluster, "Elements Remaining"=w304:u32)  [unwired: 1 in, 1 out]
            n72 = xnode "Invoke Method"("FPGA VI Reference In"=w303, "error in"=w300, "Number of Elements"=w304) -> ("error out"=w301:errorcluster)  [unwired: 1 in, 3 out]
          }
          frame True {
            n73 = xnode "Invoke Method"("FPGA VI Reference In"=w326, "error in"=w327, "Number of Elements"=u32 512, "Timeout (ms)"=-1) -> ("FPGA VI Reference Out"=w323:refnum<k20>, "error out"=w324:errorcluster, "Data"=w329:fxp<+,44,44>[])  [unwired: 1 out]
            n74 = To Double Precision Float(number=w329) -> (double precision float=w328:dbl[])
            n75 = Square Root(x=w328) -> (sqrt(x)=w321:dbl[])
            n76 = Split 1D Array(array=w321, index=256) -> (first subarray=w319:dbl[], second subarray=w318:dbl[])
            "First FFT (bin)" <- w319
            "Second FFT (bin)" <- w318
            n77 = xnode "Invoke Method"("FPGA VI Reference In"=w323, "error in"=w324, "Number of Elements"=u32 0) -> ("error out"=w325:errorcluster)  [unwired: 1 in, 3 out]
            n78 = call "Distance-Velocity Calculation RT.vi"("First FFT"=w319, "Second FFT"=w318, "Windowing"=w309, "first FFT bin"=w312, "Sample Rate (S/s)"=w307, "last FFT bin"=w313) -> ("F_rise"=→"f_rise":dbl, "maxbin_firstFFT"=→"maxbin_firstFFT":i32, "maxbin_secondFFT"=→"maxbin_secondFFT":i32, "Distance (m)"=→"Distance (m)":dbl, "f_mean"=→"f_mean":dbl, "F_fall"=→"f_fall":dbl, "Velocity (m/s)"=→"Velocity (m/s)":dbl)  [unwired: 7 in]
          }
        }
      }
      frame #2 {
        n79 = case shown="True" w337 {
          tunnel: w334 -> [w340 w344]
          tunnel: [w340 w345] -> w333
          tunnel: w332 -> [_ w341]
          frame False {
          }
          frame True {
            n80 = Decrement(x=w341) -> (x-1=w342:i32)
            n81 = Greater Or Equal?(x=w344, y=w342) -> (x >= y?=w343:bool)
            n82 = case shown="True" w343 {
              tunnel: w344 -> [w346 _]
              tunnel: [w347 0] -> w345
              frame False {
                n83 = Increment(x=w346) -> (x+1=w347:i32)
              }
              frame True {
                n84 = property class="Bool (strict)"("Value"=TRUE ("Snapshot")) -> ()  [unwired: 2 in, 2 out]
              }
            }
          }
        }
      }
    }
    n85 = node-c288() -> ()  [unwired: 1 in, 1 out]
  }
  n86 = node-c288(w40) -> ()  [unwired: 1 out]
  n87 = RT FIFO Delete(0:w20, 3:w19) -> (11:w18:errorcluster)  [unwired: 1 in]
  n88 = Merge Errors(w37, w38, w23, w18) -> (w21:errorcluster)
  n89 = flat-sequence {
    tunnel: w21 -> [w353]
    tunnel: w32 -> [w350]
    frame #0 {
      n90 = property class="Bool (strict)"(error in=w353, "Value"=FALSE ("stop")) -> (error out=w352:errorcluster)  [unwired: 1 in, 1 out]
      n91 = xnode "Invoke Method"("FPGA VI Reference In"=w350, "error in"=w352) -> ("FPGA VI Reference Out"=w355:refnum<k20>, "error out"=w354:errorcluster)
      n92 = xnode "Invoke Method"("FPGA VI Reference In"=w355, "error in"=w354) -> ("FPGA VI Reference Out"=w356:refnum<k20>, "error out"=w357:errorcluster)
      n93 = xnode "Close FPGA VI Reference"("FPGA VI Reference In"=w356, "error in"=w357) -> ()  [unwired: 1 out]
    }
  }
